vi "Test_ConstructTransport_BadFormatString_Error.vi"(8 "error in (no error)":errorcluster, 11 "TestCase in":refnum<class "TestFormattedStringBinding.lvclass">) -> (0 "error out":errorcluster, 3 "TestCase out":refnum<class "TestFormattedStringBinding.lvclass">)   [LabVIEW 2017, in "TestFormattedStringBinding.lvclass"]
uses:
  TestFormattedStringBinding.lvclass
  Source/Concrete/FormattedStringBinding/FormattedStringBinding.lvclass/FormattedStringBinding.ctl
  Source/Concrete/FormattedStringBinding/FormattedStringBinding.lvclass
  C:/Git/composed-transport/Source/Concrete/TerminalValueBinding/TerminalValueBinding.lvclass
  <vilib>/Utility/error.llb/Error Cluster From Error Code.vi
  Source/Concrete/TerminalValueBinding/Construct Terminal Value Binding.vi
panel:
  out "Return Error":errorcluster
  in  "String":string
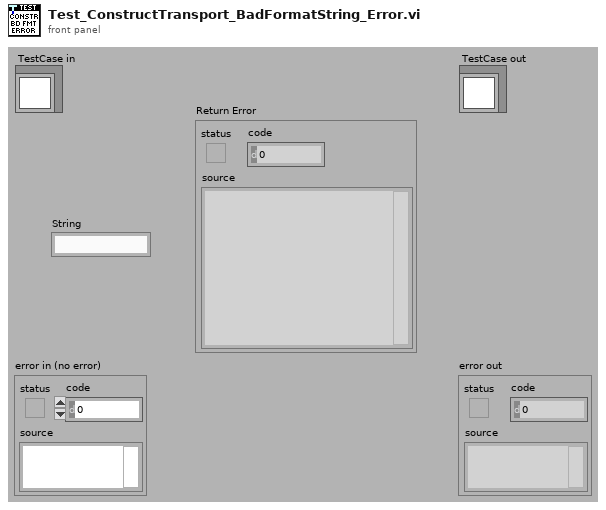
[diagram p1: front panel]
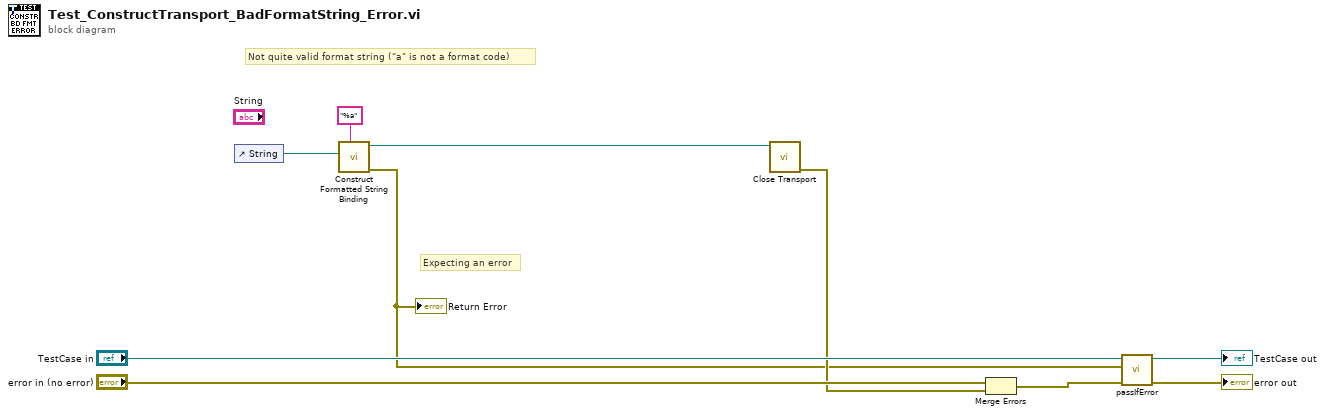
[diagram p0: block diagram]
diagram:
  # "Expecting an error"
  # "Not quite valid format string (\"a\" is not a format code)"
  n1 = control-ref of="String"() -> (w5:refnum<vi>)
  n2 = call "Construct Formatted String Binding.vi"("Format String"="%a", "Str Refnum"=w5) -> ("error out"=w1:errorcluster, "FormattedStringBinding"=w2:refnum<class "FormattedStringBinding.lvclass">)  [unwired: 8 in]
  "Return Error" <- w1
  n3 = call-dynamic "Close Transport.vi"("ITransport in"=w2) -> ("error out"=w4:errorcluster)  [unwired: 10 in]
  n4 = Merge Errors("error in (no error)", w4) -> (w6:errorcluster)
  n5 = call-dynamic "passIfError.vi"("error in (no error)"=w6, "error"=w1, "TestCase in"="TestCase in") -> ("error out"=→"error out":errorcluster, "TestCase out"=→"TestCase out":refnum<class "TestFormattedStringBinding.lvclass">)  [unwired: 7 in]
